vi "Rohde & Schwarz VNA Read Calibration Status.vi"(7 "Rohde & Schwarz VNA":T6, 8 "error in (no error)":errorcluster, 10 "Parameters to Measure":T1[](array[typedef]) {"Channel" min=1 max=99 step=1; "Parameter"."Stimulus Port" min=1 step=1; "Parameter"."Response Port" min=1 step=1}, 11 "VISA Resource Name":refnum<visa-resource-name>) -> (0 "error out":errorcluster {"code" format="%.0x"}, 1 "Parameters to Measure":T1[](array[typedef]) {"Channel" min=1 max=99 step=1; "Parameter"."Stimulus Port" min=1 step=1; "Parameter"."Response Port" min=1 step=1}, 2 "Calibration Type by Parameter":T5[](array[typedef]), 3 "dup VISA Resource Name":refnum<visa-resource-name>)   [LabVIEW 2011]
doc: "This VI for the HP 8753B is used to read the calibration type.\n\n0 response\n1 response and isolation\n2 S11 1-port\n3 S22 1-port\n4 full 2-port\n5 one path 2-port\n6 no cal detected"
uses:
  TypeDefs/Rohde & Schwarz VNA Instrument Info.ctl
  tests/S Parameter/TypeDefs/SP Parameter to Measure.ctl
  tests/S Parameter/TypeDefs/SP Parameter.ctl
  tests/S Parameter/TypeDefs/SP Calibration State.ctl
  tests/S Parameter/TypeDefs/SP Measurement Format.ctl
  TypeDefs/Rohde & Schwarz VNA Calibration State.ctl
  TypeDefs/Rohde & Schwarz VNA Conversion.ctl
  TypeDefs/Rohde & Schwarz VNA Measurement.ctl
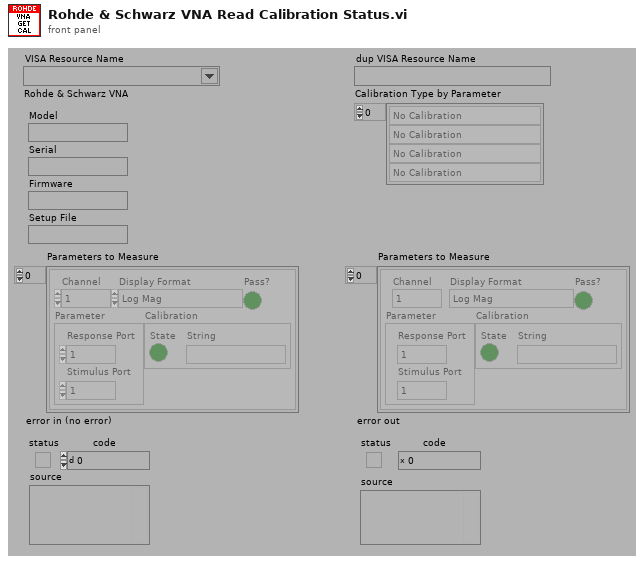
[diagram p1: front panel]
types:
  T1 = typedef "SP Parameter to Measure.ctl" = cluster{"Channel":i8, "Parameter":T2, "Calibration":T3, "Display Format":T4, "Pass?":bool}
  T2 = typedef "SP Parameter.ctl" = cluster{"Stimulus Port":i8, "Response Port":i8}
  T3 = typedef "SP Calibration State.ctl" = cluster{"State":bool, "String":string}
  T4 = typedef "SP Measurement Format.ctl" = enum32{"Log Mag", "Phase", "Delay", "Smith (R+jX)", "Polar (Re/Im)", "Linear Mag", "SWR", "Real", "Imaginary", "Smith (Lin/Phase)", "Smith (Log/Phase)", "Smith (Real/Imag)", "Smith (G+jB)", "Polar (Lin/Phase)", "Polar (Log/Phase)", "Expanded Phase", "Positive Phase", "Inverted Smith", "Unwrapped Phase", "Power Out", "Power In", "Linear Mag/Phase", "Log Mag/Phase", "Real/Imaginary"}
  T5 = typedef "Rohde & Schwarz VNA Calibration State.ctl" = enum32{"No Calibration", "Response", "Response and Isolation", "Full 1-Port (Port 1)", "Full 1-Port (Port 2)", "Full 2-Port", "One Path 2-Port", "TRL/LRM  2-Port", "TOSM Multi-Port", "TOM 2-Port", "TRM 2-Port", "TNA 2-Port"}
  T6 = typedef "Rohde & Schwarz VNA Instrument Info.ctl" = cluster{"Model":string, "Serial":string, "Firmware":string, "Setup File":string}
  T7 = typedef "Rohde & Schwarz VNA Conversion.ctl" = enum16{"Off", "Fundamental", "Harmonic", "2nd Harmonic", "3rd Harmonic", "Mixer"}
  T8 = typedef "Rohde & Schwarz VNA Measurement.ctl" = enum32{"S11", "S12", "S21", "S22", "A1 Port 1 Source", "A1 Port 2 Source", "A2 Port 1 Source", "A2 Port 2 Source", "B1 Port 1 Source", "B1 Port 2 Source", "B2 Port 1 Source", "B2 Port 2 Source", "A1/A2 Port 1 Source", "A1/A2 Port 2 Source", "A1/B1 Port 1 Source", "A1/B1 Port 2 Source", "A1/B2 Port 1 Source", "A1/B2 Port 2 Source", "A2/A1 Port 1 Source", "A2/A1 Port 2 Source", "A2/B1 Port 1 Source", "A2/B1 Port 2 Source", "A2/B2 Port 1 Source", "A2/B2 Port 2 Source", "B1/A1 Port 1 Source", "B1/A1 Port 2 Source", "B1/A2 Port 1 Source", "B1/A2 Port 2 Source", "B1/B2 Port 1 Source", "B1/B2 Port 2 Source", "B2/A1 Port 1 Source", "B2/A1 Port 2 Source", "B2/A2 Port 1 Source", "B2/A2 Port 2 Source", "B2/B1 Port 1 Source", "B2/B1 Port 2 Source", "Z<-S11", "Z<-S12", "Z<-S21", "Z<-S22", "Y<-S11", "Y<-S12", "Y<-S21", "Y<-S22", "Z11", "Z12", "Z21", "Z22", "Y11", "Y12", "Y21", "Y22", "DC±1V", "DC±10V", "Unsupported"}
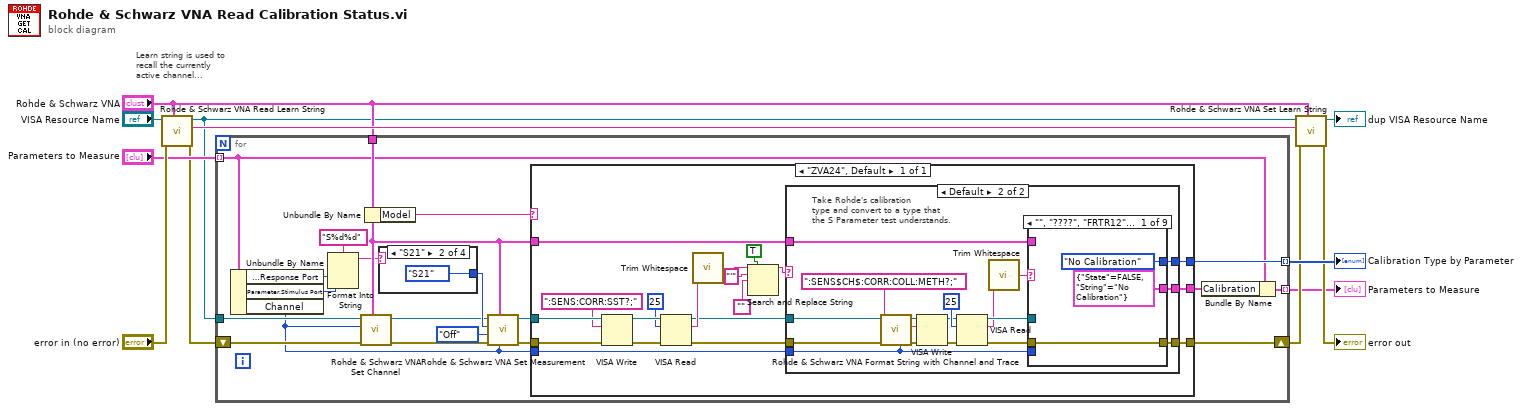
[diagram p0: block diagram]
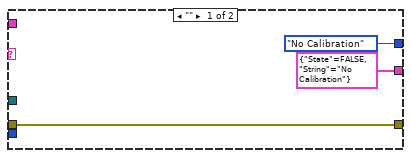
[diagram p2: hidden frame]
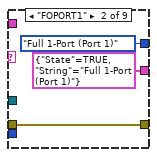
[diagram p3: hidden frame]
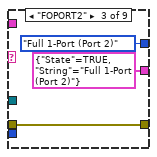
[diagram p4: hidden frame]
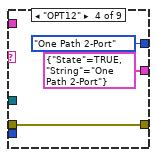
[diagram p5: hidden frame]
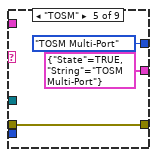
[diagram p6: hidden frame]
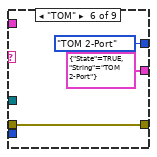
[diagram p7: hidden frame]
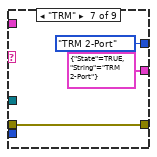
[diagram p8: hidden frame]
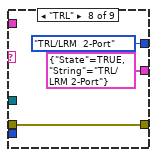
[diagram p9: hidden frame]
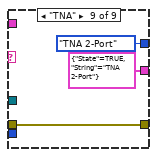
[diagram p10: hidden frame]
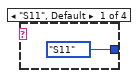
[diagram p11: hidden frame]
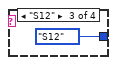
[diagram p12: hidden frame]
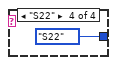
[diagram p13: hidden frame]
diagram:
  # "Learn string is used to\nrecall the currently \nactive channel..."
  n1 = call "Rohde & Schwarz VNA Read Learn String.vi"("Rohde & Schwarz VNA"="Rohde & Schwarz VNA", "error in (no error)"="error in (no error)", "VISA Resource Name"="VISA Resource Name") -> ("error out"=w3:errorcluster, "Learn String"=w10:string, "dup VISA Resource Name"=w2:refnum<visa-resource-name>)  [unwired: 6 out]
  n2 = for {
    tunnel: w2 -> [w27]
    shift-right: [w30] -> w8
    shift-left: w3 -> [w24]
    tunnel: "Parameters to Measure" -> [w15] mode=indexing
    tunnel: [w29] -> w9 mode=indexing
    tunnel: "Rohde & Schwarz VNA" -> [w21]
    tunnel: [w13] -> w1 mode=indexing
    n3 = Unbundle By Name(w15) -> ("Parameter.Response Port"=w18:i8, "Parameter.Stimulus Port"=w19:i8, "Channel"=w23:i8)
    n4 = Format Into String(format string="S%d%d", w18, w19) -> (resulting string=w16:string)  [unwired: 2 in, 1 out]
    n5 = call "Rohde & Schwarz VNA Set Channel.vi"("Rohde & Schwarz VNA"=w21, "error in (no error)"=w24, "Channel"=w23, "VISA Resource Name"=w27) -> ("error out"=w25:errorcluster, "dup VISA Resource Name"=w26:refnum<visa-resource-name>)  [unwired: 6 out]
    n6 = Unbundle By Name(w21) -> ("Model"=w20:string)
    n7 = case shown="\"S21\"" w16 {
      tunnel: [Rohde_&_Schwarz_VNA_Measurement."S11" ("Measurement (S11 - A/R)") Rohde_&_Schwarz_VNA_Measurement."S21" ("Measurement (S11 - A/R)") Rohde_&_Schwarz_VNA_Measurement."S12" ("Measurement (S11 - A/R)") Rohde_&_Schwarz_VNA_Measurement."S22" ("Measurement (S11 - A/R)")] -> w28
      frame "S11", Default {
      }
      frame "S21" {
      }
      frame "S12" {
      }
      frame "S22" {
      }
    }
    n8 = call "Rohde & Schwarz VNA Set Measurement.vi"("Channel"=w23, "Rohde & Schwarz VNA"=w21, "error in (no error)"=w25, "Conversion (Off)"=Rohde_&_Schwarz_VNA_Conversion."Off", "Measurement (S11)"=w28, "VISA Resource Name"=w26) -> ("error out"=w32:errorcluster, "dup VISA Resource Name"=w31:refnum<visa-resource-name>)  [unwired: 4 out]
    n9 = case shown="\"ZVA24\", Default" w20 {
      tunnel: w32 -> [w43]
      tunnel: w31 -> [w44]
      tunnel: [w50] -> w30
      tunnel: [w51] -> w29
      tunnel: w23 -> [w40]
      tunnel: w21 -> [w49]
      tunnel: [w33] -> w14
      frame "ZVA24", Default {
        n10 = VISA Write(VISA resource name=w44, write buffer=":SENS:CORR:SST?;" ("String"), error in (no error)=w43) -> (VISA resource name out=w46:refnum<visa-resource-name>, error out=w47:errorcluster)  [unwired: 1 out]
        n11 = VISA Read(VISA resource name=w46, byte count=u32 25, error in (no error)=w47) -> (VISA resource name out=w42:refnum<visa-resource-name>, read buffer=w48:string, error out=w41:errorcluster)  [unwired: 1 out]
        n12 = call <vilib>:"Trim Whitespace.vi"("string"=w48) -> ("trimmed string"=w38:string)  [unwired: 1 in]
        n13 = Search and Replace String(replace all?=TRUE ("replace all? (F)"), input string=w38, search string="'", replace string="") -> (result string=w35:string)  [unwired: 1 in, 6 out]
        n14 = case shown="Default" w35 {
          tunnel: [Rohde_&_Schwarz_VNA_Calibration_State."No Calibration" ("S Parameter Test Cal Type") w70] -> w51
          tunnel: w41 -> [w54 w65]
          tunnel: w42 -> [_ w64]
          tunnel: [w54 w61] -> w50
          tunnel: w49 -> [_ w59]
          tunnel: w40 -> [_ w58]
          tunnel: [T3 {"State"=FALSE, "String"="No Calibration"} w55] -> w33
          frame "" {
          }
          frame Default {
            # "Take Rohde's calibration\ntype and convert to a type that\nthe S Parameter test understands."
            n15 = call "Rohde & Schwarz VNA Format String with Channel and Trace.vi"("Trace"=w58, "String"=":SENS$CH$:CORR:COLL:METH?;") -> ("String Out"=w67:string)  [unwired: 1 in, 6 out]
            n16 = VISA Write(VISA resource name=w64, write buffer=w67, error in (no error)=w65) -> (VISA resource name out=w68:refnum<visa-resource-name>, error out=w63:errorcluster)  [unwired: 1 out]
            n17 = VISA Read(VISA resource name=w68, byte count=u32 25, error in (no error)=w63) -> (VISA resource name out=w60:refnum<visa-resource-name>, read buffer=w57:string, error out=w62:errorcluster)  [unwired: 1 out]
            n18 = call <vilib>:"Trim Whitespace.vi"("string"=w57) -> ("trimmed string"=w56:string)  [unwired: 1 in]
            n19 = case shown="\"\", \"????\", \"FRTR12\", Default" w56 {
              tunnel: [Rohde_&_Schwarz_VNA_Calibration_State."No Calibration" ("S Parameter Test Cal Type") Rohde_&_Schwarz_VNA_Calibration_State."Full 1-Port (Port 1)" ("S Parameter Test Cal Type") Rohde_&_Schwarz_VNA_Calibration_State."Full 1-Port (Port 2)" ("S Parameter Test Cal Type") Rohde_&_Schwarz_VNA_Calibration_State."One Path 2-Port" ("S Parameter Test Cal Type") Rohde_&_Schwarz_VNA_Calibration_State."TOSM Multi-Port" ("S Parameter Test Cal Type") Rohde_&_Schwarz_VNA_Calibration_State."TOM 2-Port" ("S Parameter Test Cal Type") Rohde_&_Schwarz_VNA_Calibration_State."TRM 2-Port" ("S Parameter Test Cal Type") Rohde_&_Schwarz_VNA_Calibration_State."TRL/LRM  2-Port" ("S Parameter Test Cal Type") Rohde_&_Schwarz_VNA_Calibration_State."TNA 2-Port" ("S Parameter Test Cal Type")] -> w70
              tunnel: w62 -> [w72 w75 w78 w81 w84 w87 w90 w93 w96]
              tunnel: w58 -> [_ _ _ _ _ _ _ _ _]
              tunnel: [w72 w75 w78 w81 w84 w87 w90 w93 w96] -> w61
              tunnel: w60 -> [_ _ _ _ _ _ _ _ _]
              tunnel: w59 -> [_ _ _ _ _ _ _ _ _]
              tunnel: [T3 {"State"=FALSE, "String"="No Calibration"} T3 {"State"=TRUE, "String"="Full 1-Port (Port 1)"} T3 {"State"=TRUE, "String"="Full 1-Port (Port 2)"} T3 {"State"=TRUE, "String"="One Path 2-Port"} T3 {"State"=TRUE, "String"="TOSM Multi-Port"} T3 {"State"=TRUE, "String"="TOM 2-Port"} T3 {"State"=TRUE, "String"="TRM 2-Port"} T3 {"State"=TRUE, "String"="TRL/LRM 2-Port"} T3 {"State"=TRUE, "String"="TNA 2-Port"}] -> w55
              frame "", "????", "FRTR12", Default {
              }
              frame "FOPORT1" {
              }
              frame "FOPORT2" {
              }
              frame "OPT12" {
              }
              frame "TOSM" {
              }
              frame "TOM" {
              }
              frame "TRM" {
              }
              frame "TRL" {
              }
              frame "TNA" {
              }
            }
          }
        }
      }
    }
    n20 = Bundle By Name(cluster=w15, "Calibration"=w14) -> (w13:T1)
  }
  "Calibration Type by Parameter" <- w9
  "Parameters to Measure" <- w1
  n21 = call "Rohde & Schwarz VNA Set Learn String.vi"("Rohde & Schwarz VNA"="Rohde & Schwarz VNA", "error in (no error)"=w8, "Learn String"=w10, "VISA Resource Name"=w2) -> ("error out"=→"error out":errorcluster, "dup VISA Resource Name"=→"dup VISA Resource Name":refnum<visa-resource-name>)  [unwired: 6 out]
